vi "SWaT pump control.vi"(4 "State":i16, 5 "Time":dbl format="%.2f", 6 "Sensor Values":dbl[](array[numeric]), 7 "Set Points":dbl[](array[numeric])) -> (0 "required data":T1={"Set Point names"=["Tubing size code", "L Tube Settler (mm)", "D Tube Settler (mm)", "Tube angle (degrees)", "Capture Velocity (mm/s)"], "required number of setpoints"=5, "required number of sensors"=0, "Sensor names"=[]}, 3 "output value":dbl)   [LabVIEW 2019]
panel:
  in  "pumpflow":dbl[unit][](array[numeric])=[9.549296547316535e-09, 3.342253804929783e-08, 1.2732395447351617e-07, 2.705634032562094e-07, 4.4563384065730255e-07, 6.04788783748884e-07] format="%.3f"
  in  "tubing size":enum16{"13", "14", "16", "25", "17", "18"}(ring)
  # "Enter the correct information for this control code in the required data structure below. Then make the current value default by right clicking on the border of the data structure."
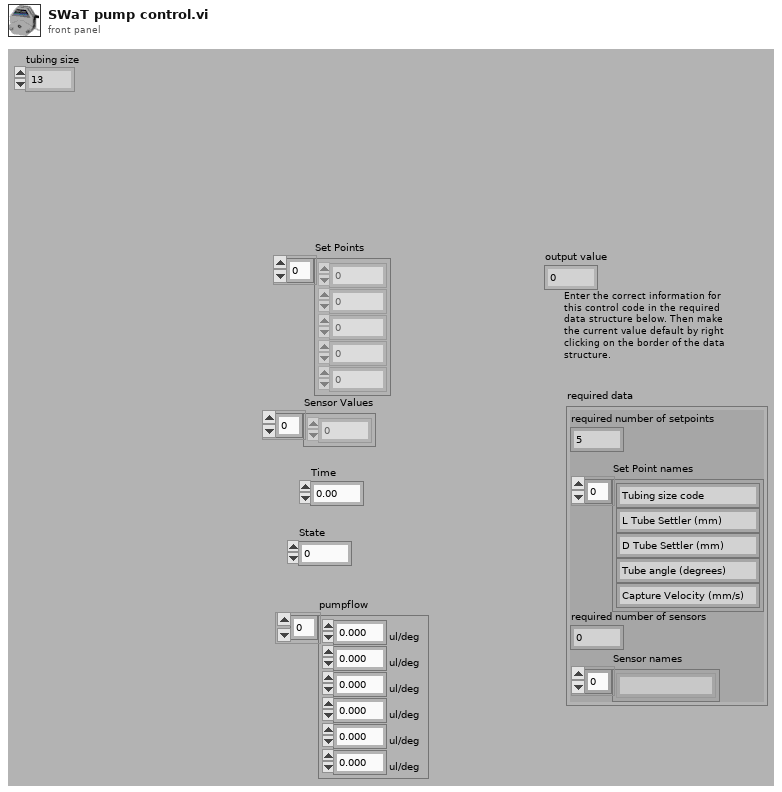
[diagram p1: front panel]
types:
  T1 = cluster{"Set Point names":string[], "required number of setpoints":u8, "required number of sensors":u8, "Sensor names":string[]}
  T2 = cluster{"Set Points[0]":dbl, "Set Points[1]":dbl, "Set Points[2]":dbl, "Set Points[3]":dbl, "Set Points[4]":dbl}
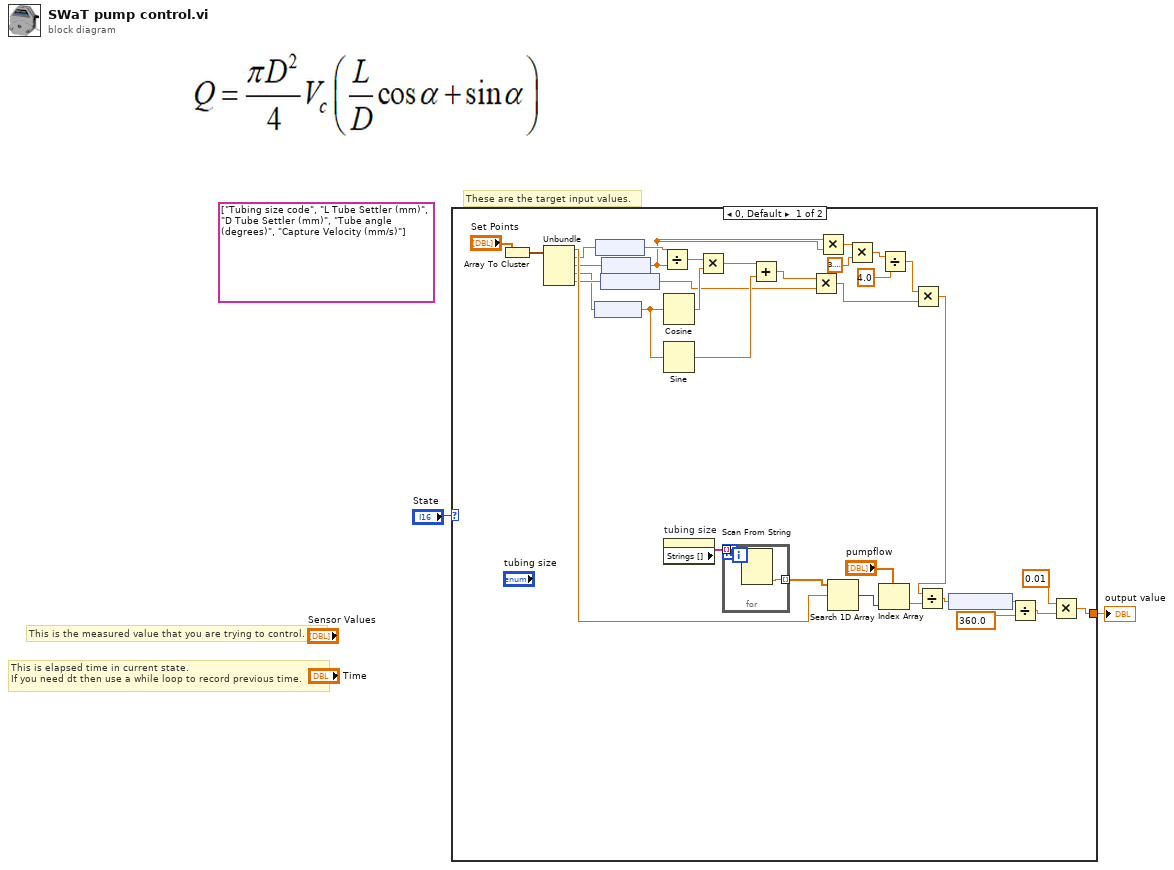
[diagram p0: block diagram]
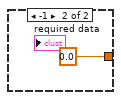
[diagram p2: hidden frame]
diagram:
  (unwired) string[] ["Tubing size code", "L Tube Settler (mm)", "D Tube Settler (mm)", "Tube angle (degrees)", "Capture Velocity (mm/s)"] ("Set Point names")
  # "These are the target input values."
  # "This is the measured value that you are trying to control."
  # "This is elapsed time in current state.\nIf you need dt then use a while loop to record previous time."
  n1 = case shown="0, Default" "State" {
    tunnel: [w31 0.0 ("fraction on")] -> w1
    frame 0, Default {
      n2 = Array To Cluster(array="Set Points") -> (cluster=w36:T2)
      n3 = Unbundle(w36) -> ("Set Points[0]"=w23:dbl, "Set Points[1]"=w15:dbl, "Set Points[2]"=w22:dbl, "Set Points[3]"=w10:dbl, "Set Points[4]"=w17:dbl)
      n4 = node(w10) -> (w9:dbl[unit])
      n5 = node(w15) -> (w4:dbl[unit])
      n6 = node(w17) -> (w8:dbl[unit])
      n7 = node(w22) -> (w3:dbl[unit])
      n8 = Divide(x=w4, y=w3) -> (x/y=w21:dbl)
      n9 = Cosine(x=w9) -> (cos(x)=w20:dbl)
      n10 = Sine(x=w9) -> (sin(x)=w18:dbl)
      n11 = property on="tubing size" class="Enum (strict)"() -> ("Strings []"=w32:string[])  [unwired: 2 in, 2 out]
      n12 = Multiply(x=w21, y=w20) -> (x*y=w19:dbl)
      n13 = for {
        tunnel: w32 -> [w38] mode=indexing
        tunnel: [w37] -> w35 mode=indexing
        n14 = Scan From String(input string=w38) -> (output 1=w37:dbl)  [unwired: 4 in, 3 out]
      }
      n15 = Add(x=w19, y=w18) -> (x+y=w16:dbl)
      n16 = Multiply(x=w16, y=w8) -> (x*y=w6:dbl[unit])
      n17 = Multiply(x=w3, y=w3) -> (x*y=w14:dbl[unit])
      n18 = Search 1D Array(1D array=w35, element=w23) -> (index of element=w24:i32)  [unwired: 1 in]
      n19 = Multiply(x=w14, y=3.141592653589793) -> (x*y=w12:dbl[unit])
      n20 = Index Array(array="pumpflow", index=w24) -> (element=w29:dbl[unit])
      n21 = Divide(x=w12, y=4.0) -> (x/y=w7:dbl[unit])
      n22 = Multiply(x=w7, y=w6) -> (x*y=w5:dbl[unit])
      n23 = Divide(x=w5, y=w29) -> (x/y=w28:dbl[unit])
      n24 = node(w28) -> (w27:dbl)
      n25 = Divide(x=w27, y=360.0) -> (x/y=w25:dbl)
      n26 = Multiply(x=0.01, y=w25) -> (x*y=w31:dbl)
    }
    frame -1 {
    }
  }
  "output value" <- w1
